vi "Set Current State.vi"(10 "State Types":T1, 11 "Model in":refnum<class "Model.lvclass">) -> (3 "Model out":refnum<class "Model.lvclass">)   [LabVIEW 2016, in "Model.lvclass"]
uses:
  Model.lvclass
  Typedefs/StateTypes.ctl
  Model.lvclass/Model.ctl
  Typedefs/HPMT_Typedefs.lvlib
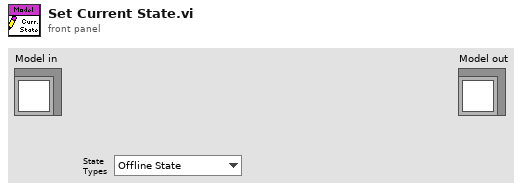
[diagram p1: front panel]
types:
  T1 = typedef "HPMT_Typedefs.lvlib/StateTypes.ctl" = enum16{"Offline State", "Fault State", "Standby State", "Disabled State", "Enabled State", "Wait For User Input State", "Test Actuator State"}
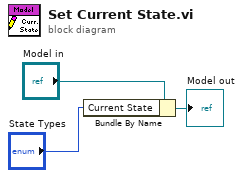
[diagram p0: block diagram]
diagram:
  n1 = Bundle By Name(cluster="Model in", "Current State"="State Types") -> (→"Model out":refnum<class "Model.lvclass">)
